vi "RobotCommand.vi"(8 "Robot Motors":T1) -> (10 "HandsMotorCmd":dbl(graph), 11 "LeftArmMotorCmd":dbl(graph), 12 "SqueezeMotorCmd":dbl(graph), 13 "RightArmMotorCmd":dbl(graph), 14 "Rotation":dbl(graph), 15 "ArmLiftMotorCmd":dbl(graph), 16 "Y_Axis":dbl(graph), 17 "LiftMotorCmd":dbl(graph), 18 "Left Arm Min Limit":bool, 19 "Arm Lift Min Limit":bool, 20 "X_axis":dbl(graph), 21 "Left Arm Max Limit":bool, 22 "Lift Max Limit":bool, 23 "Right Arm Max Limit":bool, 24 "Arm Lift Max Limit":bool, 25 "Right Arm Min Limit":bool, 26 "Lift Min Limit":bool)   [LabVIEW 2017]
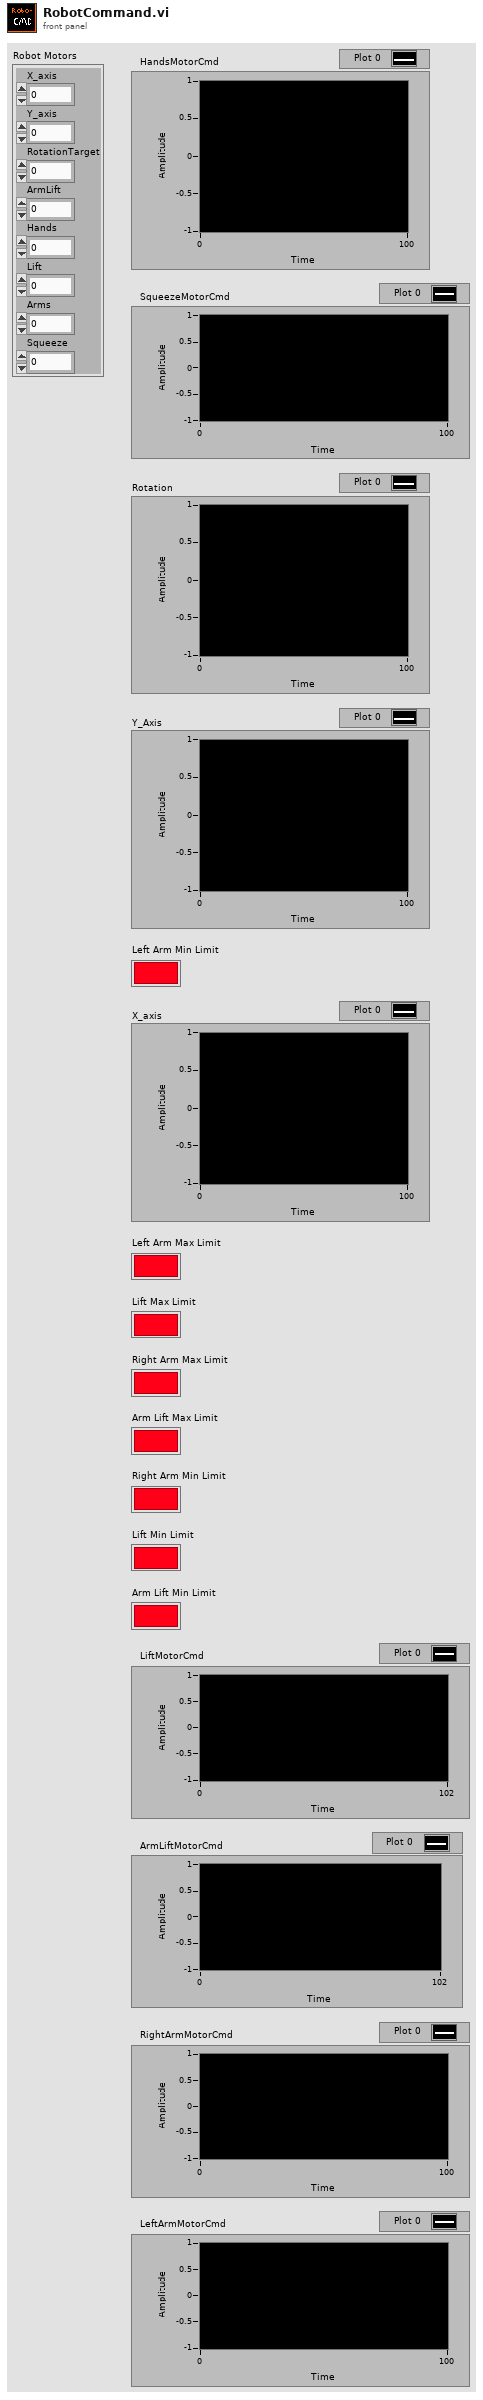
[diagram p1: front panel]
types:
  T1 = cluster{"X_axis":dbl, "Y_axis":dbl, "RotationTarget":dbl, "ArmLift":dbl, "Hands":dbl, "Lift":dbl, "Arms":dbl, "Squeeze":dbl}
  T2 = enum16{"initialize", "read", "write", "write all"}
  T3 = typedef "DioDisplayALB.ctl" = cluster{"DIO 0-LiftMinLimitSwitch":bool, "DIO 1-LiftMaxLimitSwitch":bool, "DIO 2-LiftArmMinLimitSwitch":bool, "DIO 3-LiftArmMaxLimitSwitch":bool, "DIO 4-RightArmMaxLimitSwitch":bool, "DIO 5-RightArmMinLimitSwitch":bool, "DIO 6-LeftArmMaxLimitSwitch":bool, "DIO 7-LeftArmMinLimitSwitch":bool, "DIO 8":bool, "DIO 9":bool}
  T4 = typedef "WPI_MotorControlDeviceRef.ctl" = cluster{"DeviceStatus":errorcluster, "Type":T5, "PWM":cluster{"PWM Channel":T6, "DeadBand":T7}, "CAN":cluster{"Device Number":u8, "SetOutput VI Ref":variant, "GetOutput VI Ref":variant, "Enable VI Ref":variant, "Disable VI Ref":variant, "Data":variant}, "Invert":bool, "DIO PWM":cluster{"PWM \"Enable\" Channel":T6, "DIOChannel":T8, "PWM Rate":dbl}}
  T5 = typedef "WPI_MotorControlType.ctl" = enum16{"PWM", "CAN", "DIO PWM"}
  T6 = typedef "FPGA_DIOPWMChannel.ctl" = enum8{"PWM 0", "PWM 1", "PWM 2", "PWM 3", "PWM 4", "PWM 5", "PWM 6", "PWM 7", "PWM 8", "PWM 9", "PWM MXP 0", "PWM MXP 1", "PWM MXP 2", "PWM MXP 3", "PWM MXP 4", "PWM MXP 5", "PWM MXP 6", "PWM MXP 7", "PWM MXP 8", "PWM MXP 9", "Invalid"}
  T7 = typedef "WPI_PWMDeadband.ctl" = cluster{"Name":string, "maxPositivePwm":i32, "minPositivePwm":i32, "centerPwm":i32, "maxNegativePwm":i32, "minNegativePwm":i32, "angularRange":u16}
  T8 = typedef "FPGA_DIOChannel.ctl" = enum8{"DIO 0", "DIO 1", "DIO 2", "DIO 3", "DIO 4", "DIO 5", "DIO 6", "DIO 7", "DIO 8", "DIO 9", "DIO MXP 0", "DIO MXP 1", "DIO MXP 2", "DIO MXP 3", "DIO MXP 4", "DIO MXP 5", "DIO MXP 6", "DIO MXP 7", "DIO MXP 8", "DIO MXP 9", "DIO MXP 10", "DIO MXP 11", "DIO MXP 12", "DIO MXP 13", "DIO MXP 14", "DIO MXP 15", "SPI Port CS1", "SPI Port CS2", "SPI Port CS3", "SPI Port MISO", "SPI Port MOSI", "Invalid"}
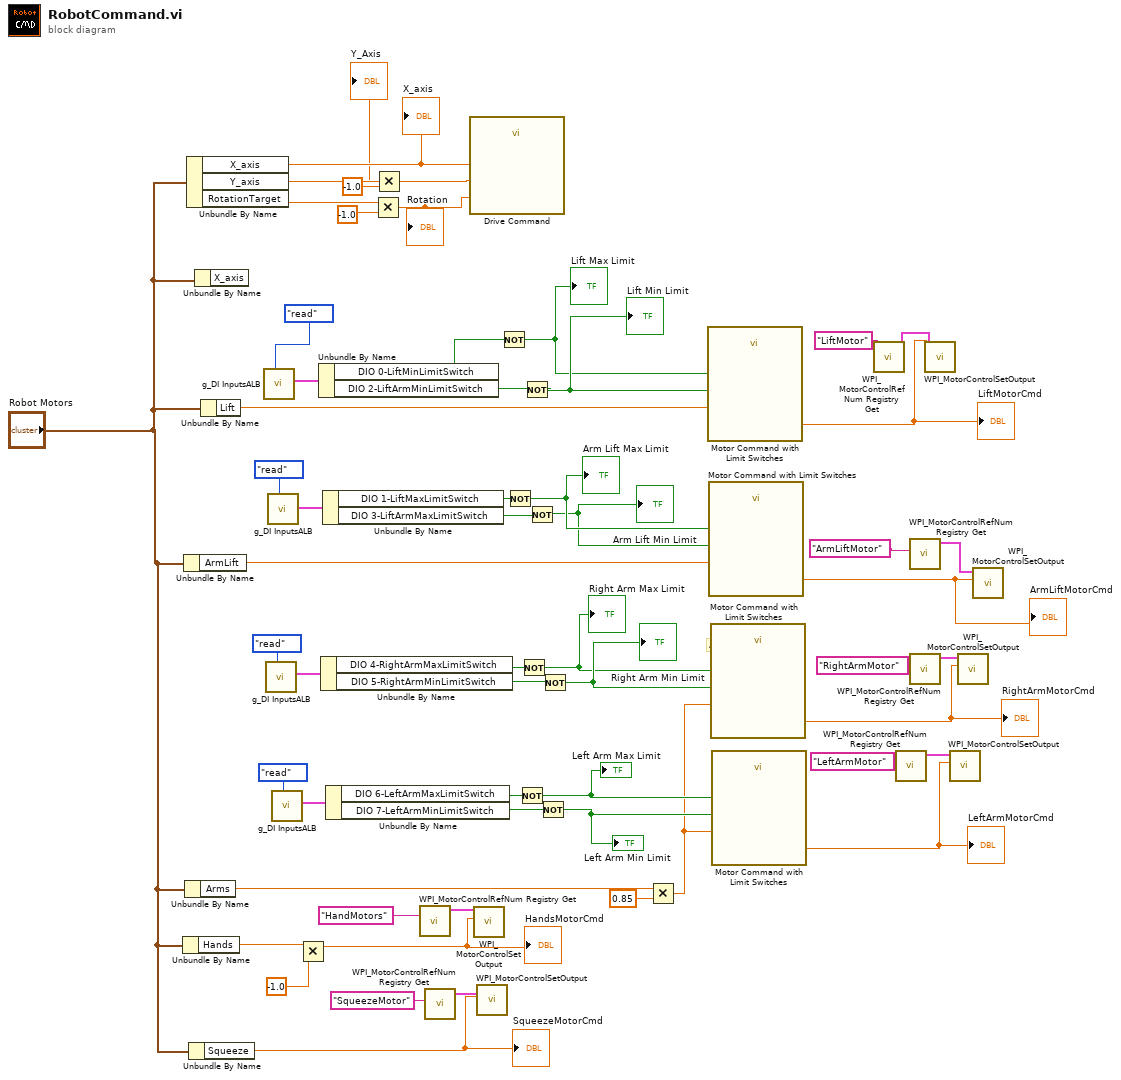
[diagram p0: block diagram]
diagram:
  # "Arms"
  n1 = Unbundle By Name("Robot Motors") -> ("Hands"=w7:dbl)
  n2 = Unbundle By Name("Robot Motors") -> ("ArmLift"=w45:dbl)
  n3 = Unbundle By Name("Robot Motors") -> ("Arms"=w24:dbl)
  n4 = Unbundle By Name("Robot Motors") -> ("X_axis"=w57:dbl, "Y_axis"=w10:dbl, "RotationTarget"=w5:dbl)
  "X_axis" <- w57
  n5 = Unbundle By Name("Robot Motors") -> ("Squeeze"=w12:dbl)
  "SqueezeMotorCmd" <- w12
  n6 = Unbundle By Name("Robot Motors") -> ()  [unwired: 1 out]
  n7 = Unbundle By Name("Robot Motors") -> ("Lift"=w14:dbl)
  n8 = call "g_DI InputsALB.vi"("Action"=T2."read") -> ("DI out"=w18:T3)  [unwired: 10 in]
  n9 = call "g_DI InputsALB.vi"("Action"=T2."read") -> ("DI out"=w27:T3)  [unwired: 10 in]
  n10 = call "g_DI InputsALB.vi"("Action"=T2."read") -> ("DI out"=w49:T3)  [unwired: 10 in]
  n11 = call "g_DI InputsALB.vi"("Action"=T2."read") -> ("DI out"=w26:T3)  [unwired: 10 in]
  n12 = Multiply(x=w7, y=-1.0) -> (x*y=w1:dbl)
  "HandsMotorCmd" <- w1
  n13 = Unbundle By Name(w18) -> ("DIO 0-LiftMinLimitSwitch"=w16:bool, "DIO 2-LiftArmMinLimitSwitch"=w15:bool)
  n14 = Unbundle By Name(w27) -> ("DIO 4-RightArmMaxLimitSwitch"=w37:bool, "DIO 5-RightArmMinLimitSwitch"=w38:bool)
  n15 = Unbundle By Name(w49) -> ("DIO 1-LiftMaxLimitSwitch"=w48:bool, "DIO 3-LiftArmMaxLimitSwitch"=w47:bool)
  n16 = Unbundle By Name(w26) -> ("DIO 6-LeftArmMaxLimitSwitch"=w39:bool, "DIO 7-LeftArmMinLimitSwitch"=w40:bool)
  n17 = Multiply(x=w5, y=-1.0) -> (x*y=w4:dbl)
  "Rotation" <- w4
  n18 = Multiply(x=w10, y=-1.0) -> (x*y=w9:dbl)
  "Y_Axis" <- w9
  n19 = call <vilib>:"WPI_MotorControlRefNum Registry Get.vi"("refnum name"="HandMotors") -> ("MotorControlDevRef"=w56:T4)  [unwired: 9 in, 1 out]
  n20 = call <vilib>:"WPI_MotorControlRefNum Registry Get.vi"("refnum name"="SqueezeMotor") -> ("MotorControlDevRef"=w13:T4)  [unwired: 9 in, 1 out]
  n21 = call "Drive Command.vi"("X"=w57, "Y"=w9, "Rotation"=w4) -> ()  [unwired: 9 in]
  n22 = call <vilib>:"WPI_MotorControlSetOutput.vi"("Output"=w1, "MotorControlDevRef"=w56) -> ()  [unwired: 7 in, 3 out]
  n23 = call <vilib>:"WPI_MotorControlSetOutput.vi"("Output"=w12, "MotorControlDevRef"=w13) -> ()  [unwired: 7 in, 3 out]
  n24 = Not(x=w16) -> (.not. x?=w19:bool)
  "Lift Max Limit" <- w19
  n25 = Not(x=w48) -> (.not. x?=w52:bool)
  "Arm Lift Max Limit" <- w52
  n26 = Not(x=w39) -> (.not. x?=w31:bool)
  "Left Arm Max Limit" <- w31
  n27 = Not(x=w37) -> (.not. x?=w33:bool)
  "Right Arm Max Limit" <- w33
  n28 = Not(x=w15) -> (.not. x?=w20:bool)
  "Lift Min Limit" <- w20
  n29 = Not(x=w47) -> (.not. x?=w51:bool)
  "Arm Lift Min Limit" <- w51
  n30 = Not(x=w40) -> (.not. x?=w32:bool)
  "Left Arm Min Limit" <- w32
  n31 = Not(x=w38) -> (.not. x?=w34:bool)
  "Right Arm Min Limit" <- w34
  n32 = Multiply(x=w24, y=0.85) -> (x*y=w30:dbl)
  n33 = call "Motor Command with Limit Switches.vi"("LowLimitSwitch"=w20, "MotorCommandIn"=w14, "HighLimitSwitch"=w19) -> (0:w21:dbl)
  "LiftMotorCmd" <- w21
  n34 = call "Motor Command with Limit Switches.vi"("LowLimitSwitch"=w51, "MotorCommandIn"=w45, "HighLimitSwitch"=w52) -> (0:w46:dbl)
  "ArmLiftMotorCmd" <- w46
  n35 = call "Motor Command with Limit Switches.vi"("LowLimitSwitch"=w34, "MotorCommandIn"=w30, "HighLimitSwitch"=w33) -> (0:w36:dbl)
  "RightArmMotorCmd" <- w36
  n36 = call "Motor Command with Limit Switches.vi"("LowLimitSwitch"=w32, "MotorCommandIn"=w30, "HighLimitSwitch"=w31) -> (0:w35:dbl)
  "LeftArmMotorCmd" <- w35
  n37 = call <vilib>:"WPI_MotorControlRefNum Registry Get.vi"("refnum name"="LiftMotor") -> ("MotorControlDevRef"=w22:T4)  [unwired: 9 in, 1 out]
  n38 = call <vilib>:"WPI_MotorControlRefNum Registry Get.vi"("refnum name"="LeftArmMotor") -> ("MotorControlDevRef"=w43:T4)  [unwired: 9 in, 1 out]
  n39 = call <vilib>:"WPI_MotorControlRefNum Registry Get.vi"("refnum name"="ArmLiftMotor") -> ("MotorControlDevRef"=w53:T4)  [unwired: 9 in, 1 out]
  n40 = call <vilib>:"WPI_MotorControlRefNum Registry Get.vi"("refnum name"="RightArmMotor") -> ("MotorControlDevRef"=w44:T4)  [unwired: 9 in, 1 out]
  n41 = call <vilib>:"WPI_MotorControlSetOutput.vi"("Output"=w21, "MotorControlDevRef"=w22) -> ()  [unwired: 7 in, 3 out]
  n42 = call <vilib>:"WPI_MotorControlSetOutput.vi"("Output"=w35, "MotorControlDevRef"=w43) -> ()  [unwired: 7 in, 3 out]
  n43 = call <vilib>:"WPI_MotorControlSetOutput.vi"("Output"=w36, "MotorControlDevRef"=w44) -> ()  [unwired: 7 in, 3 out]
  n44 = call <vilib>:"WPI_MotorControlSetOutput.vi"("Output"=w46, "MotorControlDevRef"=w53) -> ()  [unwired: 7 in, 3 out]
